vi "new_curve.vi"(10 "簇":T3, 11 "子图":T1) -> (3 "子图 2":T1)   [LabVIEW 2018, in "UI.lvlib"]
uses:
  UI.lvlib
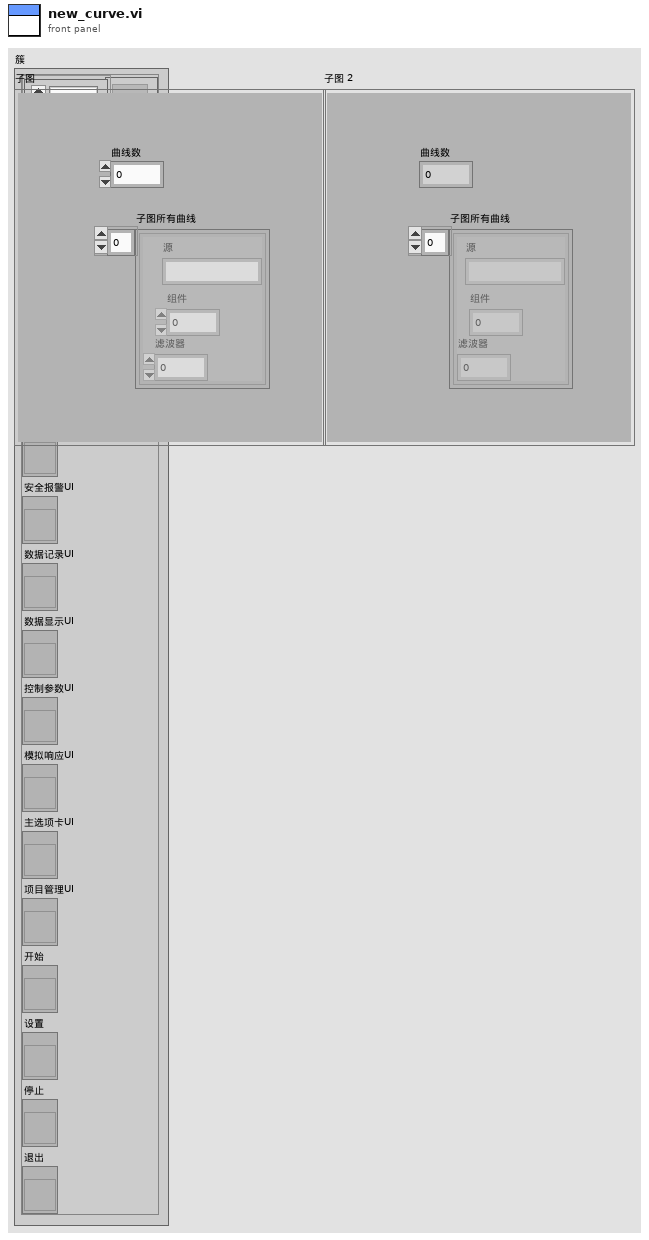
[diagram p1: front panel]
types:
  T1 = typedef "子图.ctl" = cluster{"子图所有曲线":T2[], "曲线数":u32}
  T2 = typedef "曲线簇.ctl" = cluster{"源":string, "组件":u32, "滤波器":u32}
  T3 = typedef "引用簇.ctl" = cluster{"数组":refnum<vi>[], "模拟负载UI":refnum<vi>, "波形控制UI":refnum<vi>, "模拟控制UI":refnum<vi>, "串口通信UI":refnum<vi>, "当前项目UI":refnum<vi>, "安全报警UI":refnum<vi>, "数据记录UI":refnum<vi>, "数据显示UI":refnum<vi>, "控制参数UI":refnum<vi>, "模拟响应UI":refnum<vi>, "主选项卡UI":refnum<vi>, "项目管理UI":refnum<vi>, "开始":refnum<vi>, "设置":refnum<vi>, "停止":refnum<vi>, "退出":refnum<vi>}
  T4 = enum8{"Enabled", "Disabled", "Disabled and Grayed Out"}
  T5 = typedef "组件常量.ctl" = string[]
  T6 = typedef "滤波器常量.ctl" = string[]
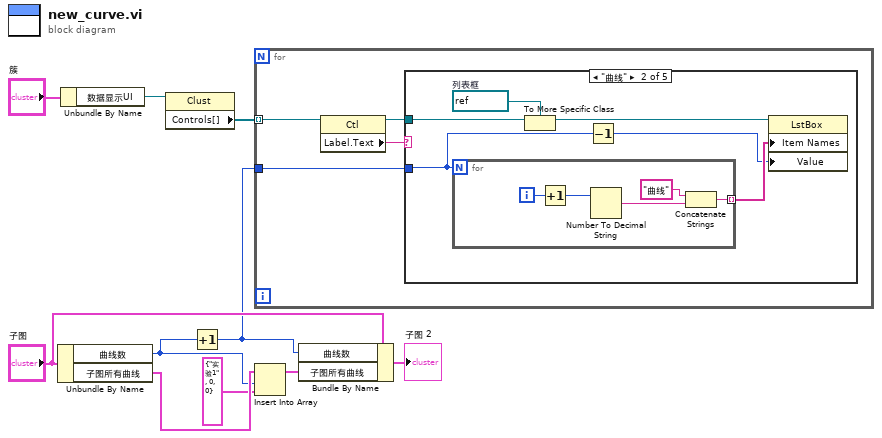
[diagram p0: block diagram]
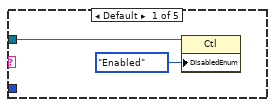
[diagram p2: hidden frame]
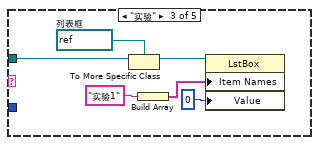
[diagram p3: hidden frame]
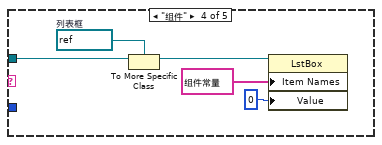
[diagram p4: hidden frame]
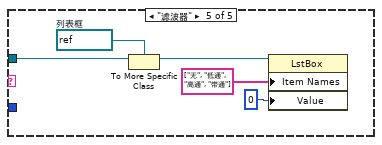
[diagram p5: hidden frame]
diagram:
  n1 = Unbundle By Name("子图") -> ("曲线数"=w5:u32, "子图所有曲线"=w6:T2[])
  n2 = Unbundle By Name("簇") -> ("数据显示UI"=w8:refnum<vi>)
  n3 = property class="Clust"(reference=w8) -> ("Controls[]"=w9:refnum<vi>[])  [unwired: 1 in, 2 out]
  n4 = Increment(x=w5) -> (x+1=w1:u32)
  n5 = for {
    tunnel: w9 -> [w14] mode=indexing
    tunnel: w1 -> [w11]
    n6 = property class="Ctl"(reference=w14) -> (reference out=w12:refnum<vi>, "Label.Text"=w13:string)  [unwired: 1 in, 1 out]
    n7 = case shown="\"曲线\"" w13 {
      tunnel: w12 -> [w16 w22 w33 w38 w43]
      tunnel: w11 -> [_ w18 _ _ _]
      frame Default {
        n8 = property class="Ctl"(reference=w16, "DisabledEnum"=T4."Enabled" ("禁用")) -> ()  [unwired: 1 in, 2 out]
      }
      frame "曲线" {
        w21 = refnum<vi> refnum  # 列表框
        n9 = for {
          N: w18 -> [_]
          tunnel: [w23] -> w19 mode=indexing
          i -> [w27]
          n10 = Increment(x=w27) -> (x+1=w26:i32)
          n11 = Number To Decimal String(number=w26) -> (decimal integer string=w24:string)  [unwired: 1 in]
          n12 = Concatenate Strings("曲线", w24) -> (w23:string)
        }
        n13 = To More Specific Class(target class=w21, reference=w22) -> (specific class reference=w20:refnum<vi>)  [unwired: 1 in, 1 out]
        n14 = Decrement(x=w18) -> (x-1=w17:u32)
        n15 = property class="LstBox"(reference=w20, "Item Names"=w19, "Value"=w17) -> ()  [unwired: 1 in, 2 out]
      }
      frame "实验" {
        w32 = refnum<vi> refnum  # 列表框
        n16 = To More Specific Class(target class=w32, reference=w33) -> (specific class reference=w31:refnum<vi>)  [unwired: 1 in, 1 out]
        n17 = Build Array("实验1") -> (w30:string[])
        n18 = property class="LstBox"(reference=w31, "Item Names"=w30, "Value"=0) -> ()  [unwired: 1 in, 2 out]
      }
      frame "组件" {
        w37 = refnum<vi> refnum  # 列表框
        n19 = To More Specific Class(target class=w37, reference=w38) -> (specific class reference=w36:refnum<vi>)  [unwired: 1 in, 1 out]
        n20 = property class="LstBox"(reference=w36, "Item Names"=T5 ["正弦", "方波", "三角", "锯齿"] ("数组"), "Value"=0) -> ()  [unwired: 1 in, 2 out]
      }
      frame "滤波器" {
        w42 = refnum<vi> refnum  # 列表框
        n21 = To More Specific Class(target class=w42, reference=w43) -> (specific class reference=w41:refnum<vi>)  [unwired: 1 in, 1 out]
        n22 = property class="LstBox"(reference=w41, "Item Names"=T6 ["无", "低通", "高通", "带通"] ("数组"), "Value"=0) -> ()  [unwired: 1 in, 2 out]
      }
    }
  }
  n23 = Insert Into Array(array=w6, index=w5, new element=T2 {"源"="实验1", "组件"=0, "滤波器"=0} ("新元素/子数组")) -> (w3:T2[])
  n24 = Bundle By Name(cluster="子图", "曲线数"=w1, "子图所有曲线"=w3) -> (→"子图 2":T1)
